vi "emi_FP Activate.vi"(5 "VI Refnum(This vi)":refnum<vi>, 7 "Hidden(F)":bool, 9 "error in (no error)":errorcluster) -> (6 "VI Refnum":refnum<vi>, 10 "error out":errorcluster)   [LabVIEW 2010]
doc: "Describe...\n\n\nIf no VI ref in, then the VI containing this VI is used.\nIf VI has multiple panes, only the first pane will be used.\n\nOn error in: Does not run."
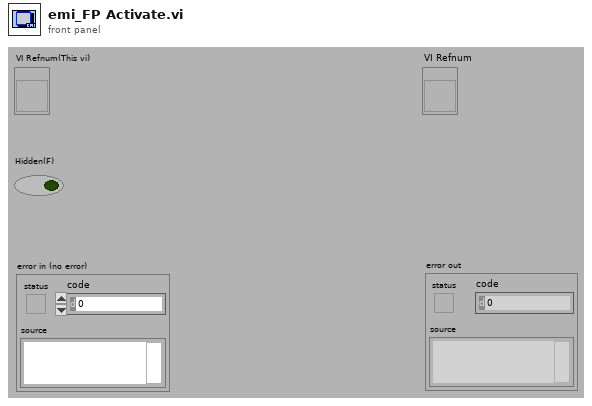
[diagram p1: front panel]
types:
  T1 = enum32{"Invalid", "Standard", "Closed", "Hidden", "Minimized", "Maximized"}
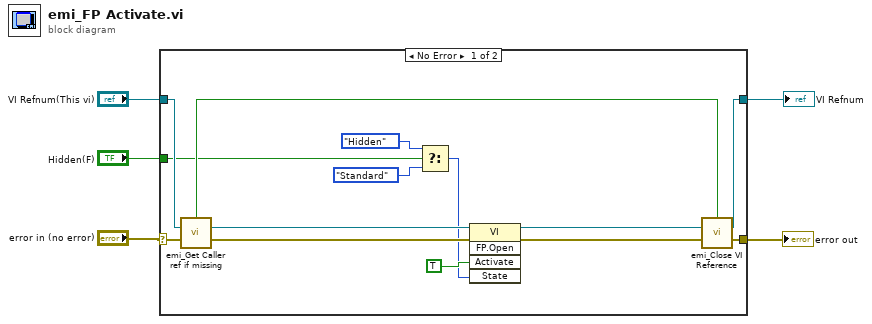
[diagram p0: block diagram]
diagram:
  n1 = case shown="No Error" "error in (no error)" {
    selector: "error in (no error)" -> [w18 w21]
    tunnel: [w16 w21] -> w5
    tunnel: "VI Refnum(This vi)" -> [w17 w20]
    tunnel: [w15 w20] -> w3
    tunnel: "Hidden(F)" -> [w7 _]
    frame No Error {
      n2 = call "emi_Get Caller ref if missing.vi"("VI Refnum(Calling VI)"=w17, "error in (no error)"=w18) -> ("Ref Generated"=w19:bool, "VI Refnum Out"=w14:refnum<vi>, "error out"=w13:errorcluster)  [unwired: 11 in]
      n3 = Select(t=T1."Hidden" ("State"), s=w7, f=T1."Standard" ("State")) -> (s? t:f=w6:T1)
      n4 = invoke class="VI" method="FP.Open"(reference=w14, error in=w13, "Activate"=TRUE ("Activate?"), "State"=w6) -> (reference out=w11:refnum<vi>, error out=w12:errorcluster)  [unwired: 1 in, 3 out]
      n5 = call "emi_Close VI Reference.vi"("Close ref?(T)"=w19, "VI Refnum"=w11, "error in (no error)"=w12) -> ("VI Refnum Out"=w15:refnum<vi>, "error out"=w16:errorcluster)  [unwired: 11 in]
    }
    frame Error {
    }
  }
  "error out" <- w5
  "VI Refnum" <- w3
